vi "Calc - HPkw.vi"(11 "02-04-9871(Modbus)":dbl[](array[numeric])) -> (3 "HPKW":dbl)   [LabVIEW 2018, in "Controller (Host).lvlib"]
uses:
  Controller (Host).lvlib
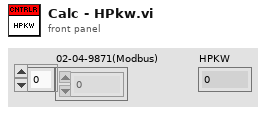
[diagram p1: front panel]
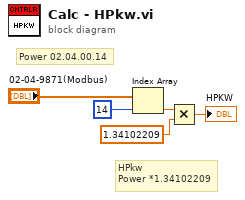
[diagram p0: block diagram]
diagram:
  # "HPkw\nPower *1.34102209"
  # "Power 02.04.00.14"
  n1 = Index Array(array="02-04-9871(Modbus)", index=14) -> (element=w5:dbl)
  n2 = Multiply(x=w5, y=1.34102209) -> (x*y=→"HPKW":dbl)
